vi "Create Edit Table of Markers.vi"(11 "markers":T1[](array[typedef])) -> (3 "Array":string[](array[string]))   [LabVIEW 2014, in "Graph Extensions.lvlib"]
uses:
  Graph Extensions.lvlib
  controls/markerType.ctl
  controls/MarkerInfo.ctl
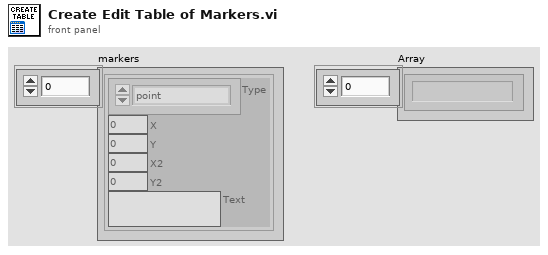
[diagram p1: front panel]
types:
  T1 = typedef "Graph Extensions.lvlib/MarkerInfo.ctl" = cluster{"Type":T2, "X":dbl, "Y":dbl, "X2":dbl, "Y2":dbl, "Text":string}
  T2 = typedef "Graph Extensions.lvlib/markerType.ctl" = enum16{"point", "arrow", "horiz", "vert", "vert range", "horiz range", "box"}
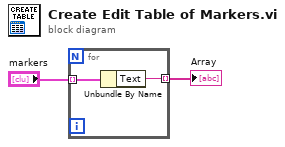
[diagram p0: block diagram]
diagram:
  n1 = for {
    tunnel: "markers" -> [w4] mode=indexing
    tunnel: [w3] -> w1 mode=indexing
    n2 = Unbundle By Name(w4) -> ("Text"=w3:string)
  }
  "Array" <- w1
